vi "sortLinesAndVolumes.vi"(7 "no new lines coming":bool, 8 "error in (no error)":errorcluster, 9 "Queues":T1, 10 "Array of lines":T2[](array[typedef])) -> (0 "error out":errorcluster, 1 "lost vol":cluster{"volume num":u32, "num lines":u32}[](array[cluster]), 2 "leftover lines":T2[](array[typedef]), 3 "last volume processed":u32, 4 "lines sorted":i32, 5 "lines lost":i32)   [LabVIEW 2010]
uses:
  line_info.ctl
  internal_queues.ctl
  volume_with_lines.ctl
  volume_info.ctl
  kalman_result_scaled.ctl
  projection buffers.ctl
  location3D.ctl
  spot location.ctl
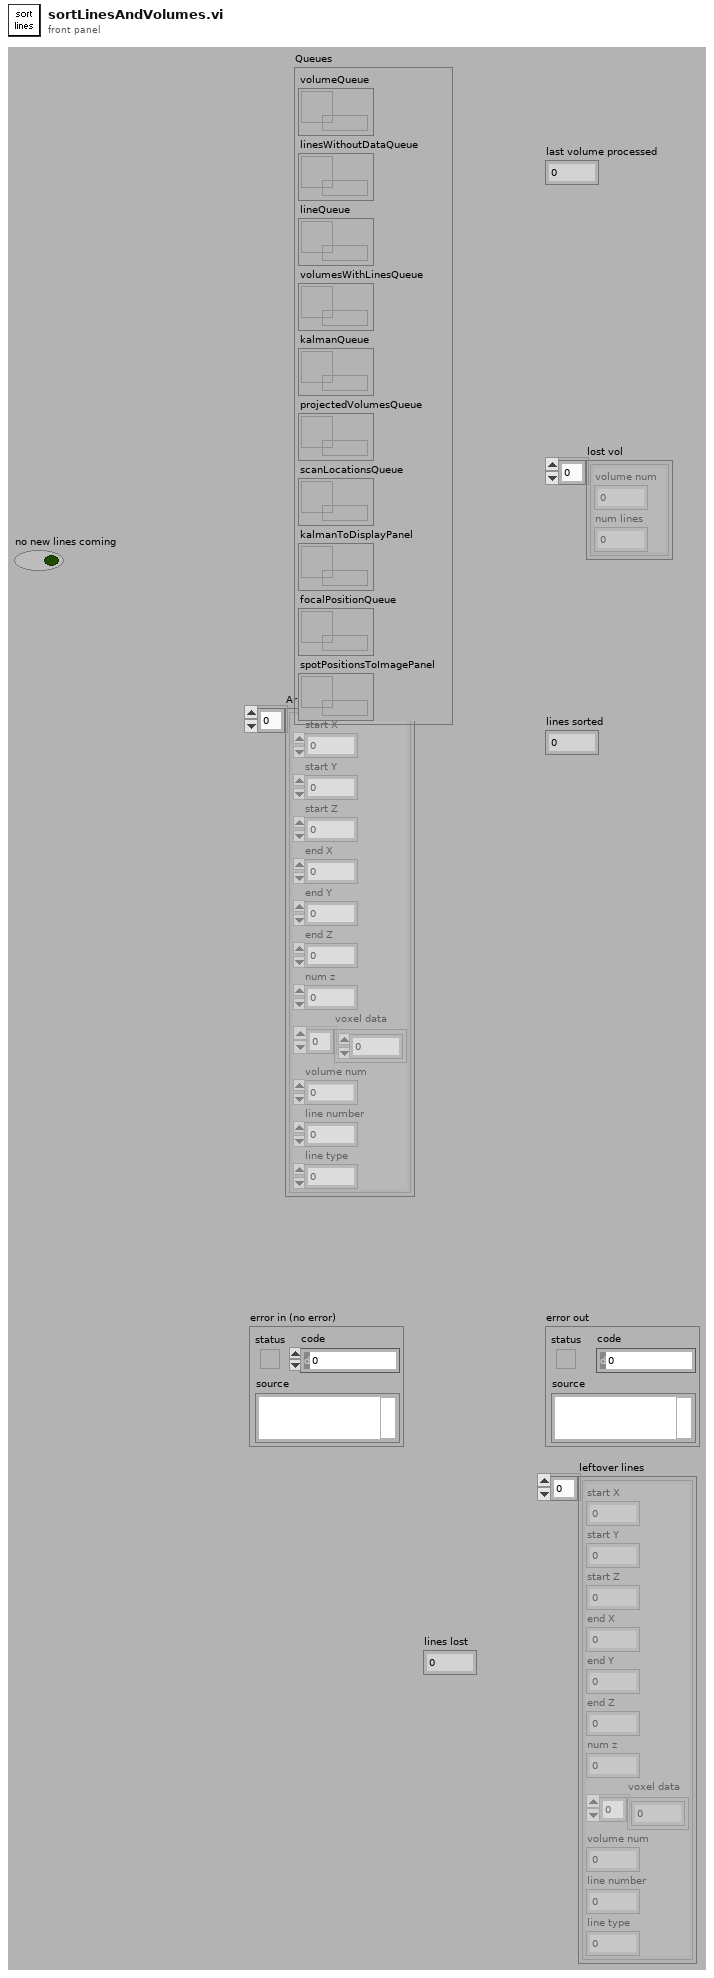
[diagram p1: front panel]
types:
  T1 = typedef "internal_queues.ctl" = cluster{"volumeQueue":refnum<queue>, "linesWithoutDataQueue":refnum<queue>, "lineQueue":refnum<queue>, "volumesWithLinesQueue":refnum<queue>, "kalmanQueue":refnum<queue>, "projectedVolumesQueue":refnum<queue>, "scanLocationsQueue":refnum<queue>, "kalmanToDisplayPanel":refnum<queue>, "focalPositionQueue":refnum<queue>, "spotPositionsToImagePanel":refnum<queue>}
  T2 = typedef "line_info.ctl" = cluster{"start X":i16, "start Y":i16, "start Z":i16, "end X":i16, "end Y":i16, "end Z":i16, "num z":u8, "voxel data":u32[], "volume num":u32, "line number":u16, "line type":u16}
  T3 = cluster{"volume num":u32, "lines":T2[], "num lines":u32}[]
  T4 = cluster{"min x":i16, "deltaX":dbl, "num x":u32, "max x":i16, "min y":i16, "deltaY":dbl, "num y":u32, "max y":i16, "num z":u32, "num voxels":u32, "voxels read":u32, "volume num":u32}
  T5 = cluster{"volume info":cluster{"min x":i16, "deltaX":dbl, "num x":u32, "max x":i16, "min y":i16, "deltaY":dbl, "num y":u32, "max y":i16, "num z":u32, "num voxels":u32, "voxels read":u32, "volume num":u32}, "lines":T2[]}
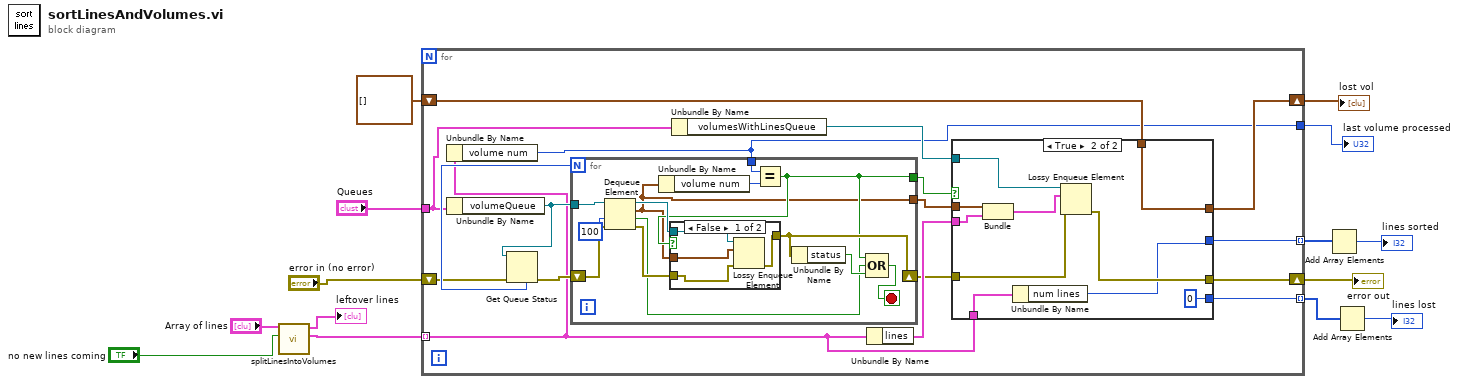
[diagram p0: block diagram]
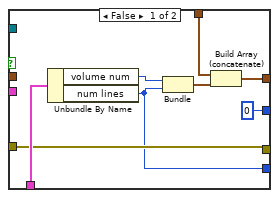
[diagram p2: hidden frame]
diagram:
  n1 = call "splitLinesIntoVolumes.vi"("don't save lines for future"="no new lines coming", "Array of lines"="Array of lines") -> ("split lines"=w12:T3, "lines for future volume"=→"leftover lines":T2[])  [unwired: 8 in]
  n2 = for {
    tunnel: w12 -> [w20] mode=indexing
    tunnel: "Queues" -> [w26]
    shift-right: [w21] -> w7
    shift-left: "error in (no error)" -> [w29]
    shift-right: [w19] -> w8
    shift-left: cluster{"volume num":u32, "num lines":i32}[] [] -> [w18]
    tunnel: [w17] -> w5 mode=indexing
    tunnel: [w16] -> w6 mode=indexing
    tunnel: [w15] -> w1
    n3 = Unbundle By Name(w20) -> ("volume num"=w15:u32)
    n4 = Unbundle By Name(w26) -> ("volumeQueue"=w31:refnum<queue>)
    n5 = Get Queue Status(queue=w31, error in (no error)=w29) -> (error out=w28:errorcluster, # elements in queue=w30:i32)  [unwired: 1 in, 6 out]
    n6 = for {
      N: w30 -> [_]
      tunnel: w31 -> [w62]
      shift-right: [w55] -> w22
      shift-left: w28 -> [w61]
      tunnel: w15 -> [w58]
      tunnel: [w52] -> w27
      tunnel: [w51] -> w24
      stop <- w50 stop-if-true
      n7 = Dequeue Element(queue=w62, timeout in ms (-1)=100, error in (no error)=w61) -> (queue out=w56:refnum<queue>, element=w51:T4, timed out?=w53:bool, error out=w57:errorcluster)
      n8 = Unbundle By Name(w51) -> ("volume num"=w59:u32)
      n9 = Equal?(x=w58, y=w59) -> (x = y?=w52:bool)
      n10 = case shown="False" w52 {
        tunnel: w57 -> [w64 w67]
        tunnel: w51 -> [w65 _]
        tunnel: w56 -> [w66 _]
        tunnel: [w63 w67] -> w55
        frame False {
          n11 = Lossy Enqueue Element(queue=w66, element=w65, error in (no error)=w64) -> (error out=w63:errorcluster)  [unwired: 3 out]
        }
        frame True {
        }
      }
      n12 = Unbundle By Name(w55) -> ("status"=w54:bool)
      n13 = Compound Arithmetic op=OR(w52, w53, w54) -> (w50:bool)
    }
    n14 = Unbundle By Name(w26) -> ("volumesWithLinesQueue"=w25:refnum<queue>)
    n15 = Unbundle By Name(w20) -> ("lines"=w23:T2[])
    n16 = case shown="True" w27 {
      tunnel: w25 -> [_ w49]
      tunnel: w23 -> [_ w47]
      tunnel: w24 -> [_ w48]
      tunnel: w22 -> [w34 w45]
      tunnel: [w34 w44] -> w21
      tunnel: w20 -> [w39 w42]
      tunnel: [w36 w43] -> w19
      tunnel: w18 -> [w35 w43]
      tunnel: [u32 0 ("num lines") w41] -> w17
      tunnel: [w33 u32 0 ("num lines")] -> w16
      frame False {
        n17 = Unbundle By Name(w39) -> ("volume num"=w38:u32, "num lines"=w33:u32)
        n18 = Bundle("volume num"=w38, "num lines"=w33) -> (w37:cluster{"volume num":u32, "num lines":u32})  [unwired: 1 in]
        n19 = Build Array (concatenate)(w35, w37) -> (w36:cluster{"volume num":u32, "num lines":u32}[])
      }
      frame True {
        n20 = Bundle("volume info"=w48, "lines"=w47) -> (w46:T5)  [unwired: 1 in]
        n21 = Unbundle By Name(w42) -> ("num lines"=w41:u32)
        n22 = Lossy Enqueue Element(queue=w49, element=w46, error in (no error)=w45) -> (error out=w44:errorcluster)  [unwired: 3 out]
      }
    }
  }
  "error out" <- w7
  "lost vol" <- w8
  "last volume processed" <- w1
  n23 = Add Array Elements(numeric array=w5) -> (sum=→"lines sorted":u32)
  n24 = Add Array Elements(numeric array=w6) -> (sum=→"lines lost":u32)
